vi "ATS_GetSDKVersion.vi"() -> (0 "Return Code":u32, 1 "SDK_#":u32 format="%09.0f", 2 "SDK_Version":string)   [LabVIEW 2014]
doc: "_____AlazarTech, Scope_____\n\nRetrieve the SDK version number which is the ATSApi version.\n\nOutput:\n\"SDK_Version\" = version in text format.\n\"SDK_#\" = version in U32 format.\n\nU32 format = (1st x 1E6) + (2nd x 1E3) + 3rd"
uses:
  ATSApi.dll
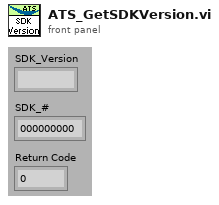
[diagram p1: front panel]
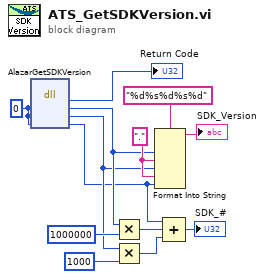
[diagram p0: block diagram]
diagram:
  w10 = u8 0
  w11 = "."
  n1 = dll-call lib="D:/IntensityOCT/trunk/ATSApi.*" fn="AlazarGetSDKVersion"(w10, w10, w10) -> (→"Return Code":u32, w4:u8, w3:u8, w2:u8)  [unwired: 3 in, 2 out]
  n2 = Multiply(x=w4, y=u32 1000000) -> (x*y=w8:u32)
  n3 = Multiply(x=w3, y=u32 1000 ("x")) -> (x*y=w7:u32)
  n4 = Format Into String(format string="%d%s%d%s%d", w4, w11, w3, w11, w2) -> (resulting string=→"SDK_Version":string)  [unwired: 2 in, 1 out]
  n5 = Compound Arithmetic op=ADD(w2, w8, w7) -> (→"SDK_#":u32)
